vi "set scan from tracking.vi"(7 "tracking?":bool, 8 "counts per cycle":u16, 9 "tracking settings":T1, 10 "tracking state in":T3, 11 "scan specification":T2) -> (2 "tracking state out":T3, 3 "scan specification out":T2)   [LabVIEW 2010]
uses:
  kalman 3-axis state.ctl
  integrating single axis kalman state.ctl
  scan_specification_tagResonant.ctl
  polar tracking settings.ctl
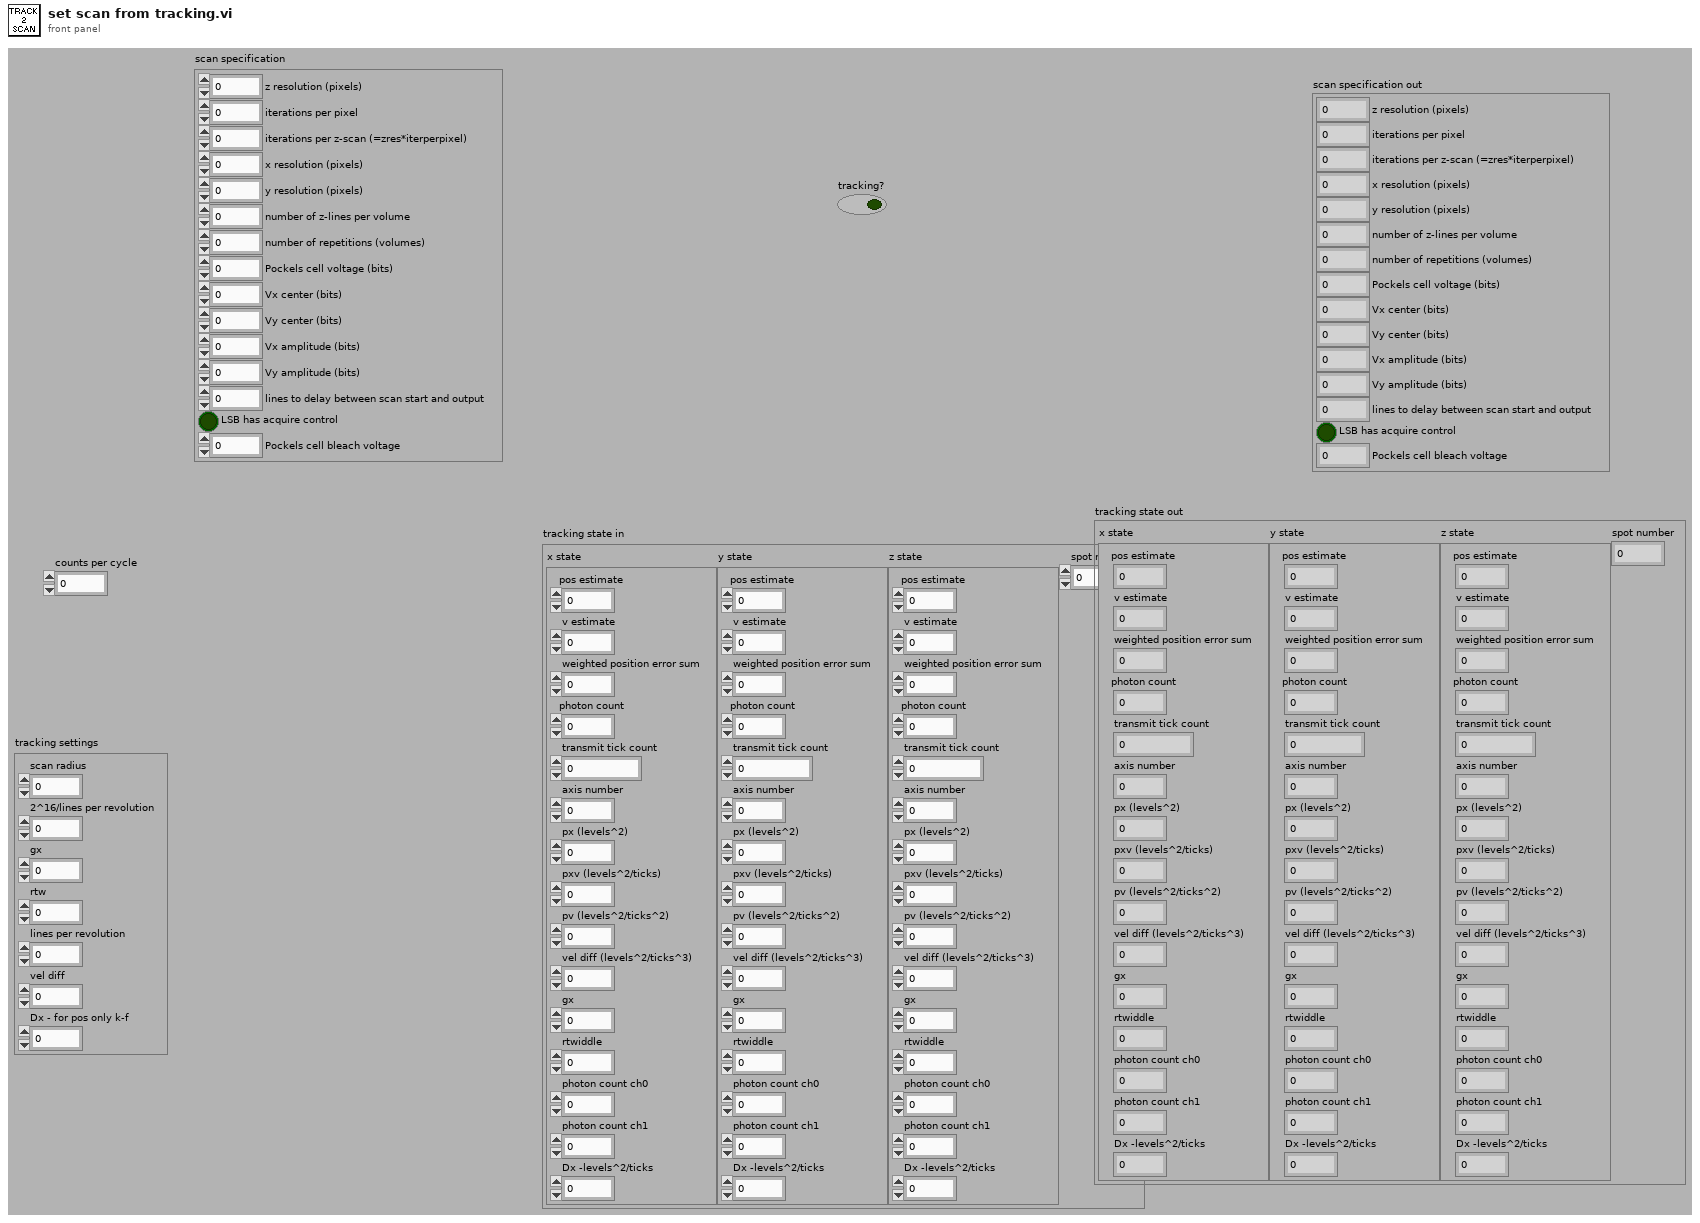
[diagram p1: front panel]
types:
  T1 = typedef "polar tracking settings.ctl" = cluster{"scan radius":u16, "2^16/lines per revolution":u16, "gx":fxp<+,16,8>, "rtw":fxp<+,16,26>, "lines per revolution":u8, "vel diff":fxp<+,24,-22>, "Dx - for pos only k-f":fxp<+,32,19>}
  T2 = typedef "scan_specification_tagResonant.ctl" = cluster{"z resolution (pixels)":u16, "iterations per pixel":u16, "iterations per z-scan (=zres*iterperpixel)":u16, "x resolution (pixels)":u16, "y resolution (pixels)":u16, "number of z-lines per volume":u16, "number of repetitions (volumes)":i32, "Pockels cell voltage (bits)":i16, "Vx center (bits)":i16, "Vy center (bits)":i16, "Vx amplitude (bits)":i16, "Vy amplitude (bits)":i16, "lines to delay between scan start and output":u16, "LSB has acquire control":bool, "Pockels cell bleach voltage":i16}
  T3 = typedef "kalman 3-axis state.ctl" = cluster{"x state":T4, "y state":T4, "z state":T4, "spot number":u8}
  T4 = typedef "integrating single axis kalman state.ctl" = cluster{"pos estimate":fxp<+/-,32,16>, "v estimate":fxp<+/-,16,0>, "weighted position error sum":fxp<+/-,32,32>, "photon count":u32, "transmit tick count":u32, "axis number":u8, "px (levels^2)":fxp<+,32,19>, "pxv (levels^2/ticks)":fxp<+,32,2>, "pv (levels^2/ticks^2)":fxp<+,32,-14>, "vel diff (levels^2/ticks^3)":fxp<+,24,-22>, "gx":fxp<+,16,8>, "rtwiddle":fxp<+,16,26>, "photon count ch0":u32, "photon count ch1":u32, "Dx -levels^2/ticks":fxp<+,32,19>}
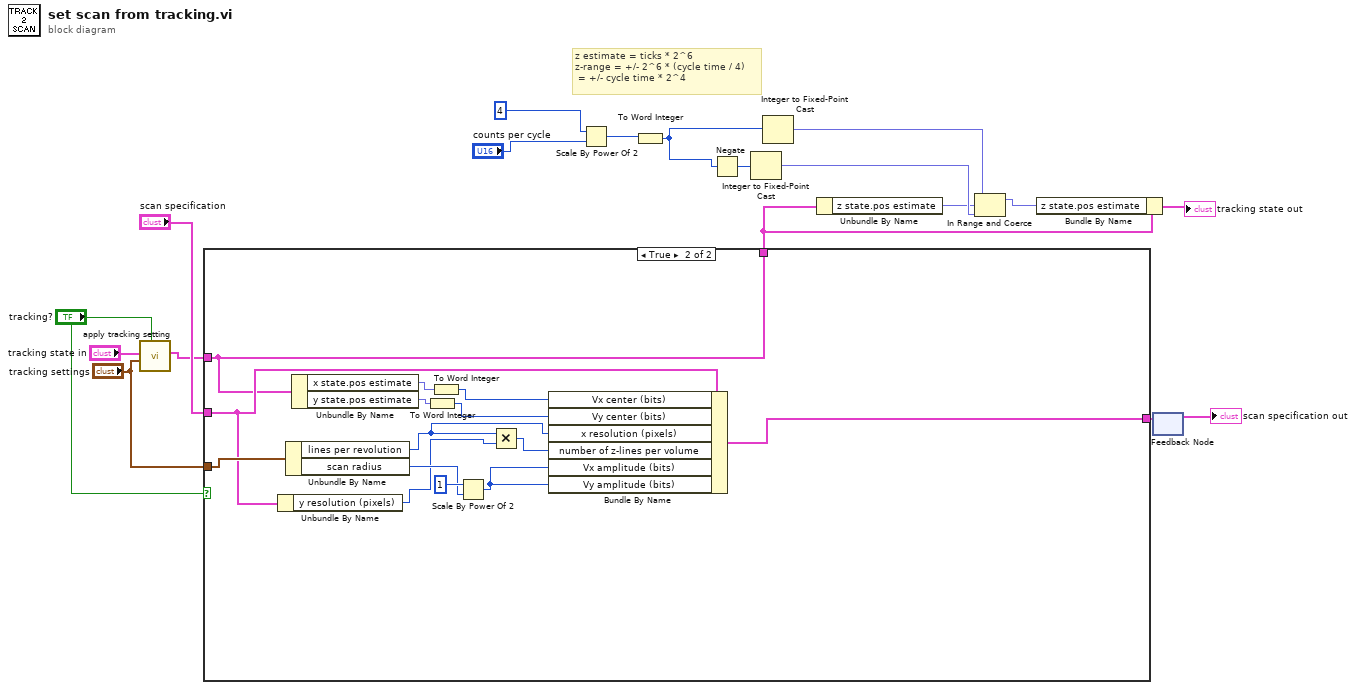
[diagram p0: block diagram]
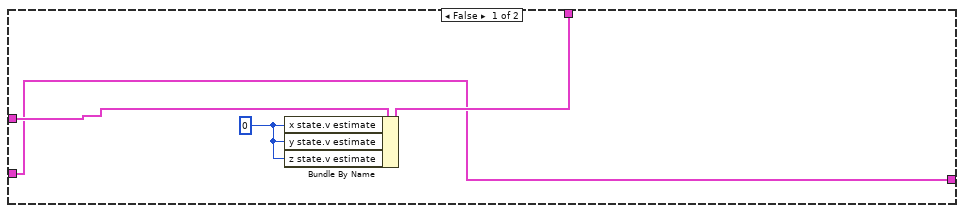
[diagram p2: hidden frame]
diagram:
  # "z estimate = ticks * 2^6\nz-range = +/- 2^6 * (cycle time / 4)\n = +/- cycle time * 2^4"
  n1 = call "apply tracking setting.vi"("tracking?"="tracking?", "tracking settings"="tracking settings", "tracking state in"="tracking state in") -> ("tracking state out"=w14:T3)  [unwired: 8 in]
  n2 = case shown="True" "tracking?" {
    tunnel: w14 -> [w22 w23]
    tunnel: "scan specification" -> [w20 w27]
    tunnel: [w21 w23] -> w2
    tunnel: [w20 w34] -> w17
    tunnel: "tracking settings" -> [_ w29]
    frame False {
      w19 = i16 0
      n3 = Bundle By Name(cluster=w22, "x state.v estimate"=w19, "y state.v estimate"=w19, "z state.v estimate"=w19) -> (w21:T3)
    }
    frame True {
      n4 = Unbundle By Name(w27) -> ("y resolution (pixels)"=w26:u16)
      n5 = Unbundle By Name(w29) -> ("lines per revolution"=w24:u8, "scan radius"=w28:u16)
      n6 = Unbundle By Name(w23) -> ("x state.pos estimate"=w33:fxp<+/-,32,16>, "y state.pos estimate"=w31:fxp<+/-,32,16>)
      n7 = To Word Integer(number=w31) -> (16bit integer=w30:i16)
      n8 = To Word Integer(number=w33) -> (16bit integer=w32:i16)
      n9 = Scale By Power Of 2(n=1, x=w28) -> (x*2^n=w35:u16)
      n10 = Multiply(x=w24, y=w26) -> (x*y=w25:u16)
      n11 = Bundle By Name(cluster=w27, "Vx center (bits)"=w32, "Vy center (bits)"=w30, "x resolution (pixels)"=w24, "number of z-lines per volume"=w25, "Vx amplitude (bits)"=w35, "Vy amplitude (bits)"=w35) -> (w34:T2)
    }
  }
  n12 = Scale By Power Of 2(n=u8 4 ("x"), x="counts per cycle") -> (x*2^n=w6:u16)
  n13 = To Word Integer(number=w6) -> (16bit integer=w4:i16)
  n14 = Negate(x=w4) -> (-x=w3:i16)
  n15 = Integer to Fixed-Point Cast(integer=w3) -> (fixed-point=w9:fxp<+/-,16,16>)  [unwired: 1 in]
  n16 = Integer to Fixed-Point Cast(integer=w4) -> (fixed-point=w10:fxp<+/-,16,16>)  [unwired: 1 in]
  n17 = Unbundle By Name(w2) -> ("z state.pos estimate"=w5:fxp<+/-,32,16>)
  n18 = In Range and Coerce(upper limit=w10, x=w5, lower limit=w9) -> (coerced(x)=w11:fxp<+/-,32,16>)  [unwired: 1 out]
  n19 = Bundle By Name(cluster=w2, "z state.pos estimate"=w11) -> (→"tracking state out":T3)
  n20 = feedback-in #1(w17) -> ()
  n21 = feedback #1() -> (→"scan specification out":T2)  [unwired: 1 in]
